vi "fgt set sensor Custom Scale Ex.vi"(8 "error in (no error)":errorcluster, 9 "SMax":sgl, 10 "Custom scale":T1, 11 "sensorIndex":u32) -> (0 "error out":errorcluster)   [LabVIEW 2020, in "fgt_SDK.lvlib"]
doc: "Apply a custom scale factor on sensor read value. This function is useful in order to adapt read sensor value to physical measurement.\nFor example if a flow-unit is used with a special oil and it's calibration table is set to H2O, read flowrate is not correct.\nScale factor is applied using following formula: scaled_value = a*sensor_value + b*sensor_value^2 + c*sensor_value^3.\nWhen applying a custom scale factor, sensor range may increase very rapidly, SMax parameter is ment to limit this maximal value.\nThis function purpose is to be used with the regulation in order to avoid too high maximum range on the sensor. Not supported by IPS."
uses:
  fgt_SDK.lvlib
  TypeDefs/fgt_SCALE.ctl
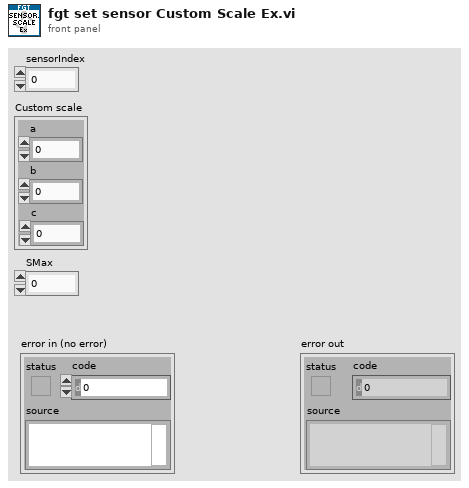
[diagram p1: front panel]
types:
  T1 = typedef "fgt_SDK.lvlib/fgt_SCALE.ctl" = cluster{"a":sgl, "b":sgl, "c":sgl}
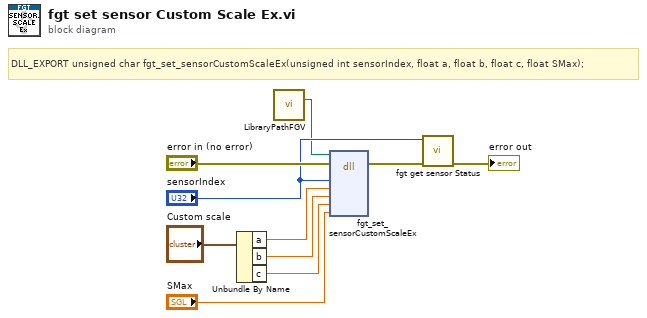
[diagram p0: block diagram]
diagram:
  # "DLL_EXPORT unsigned char fgt_set_sensorCustomScaleEx(unsigned int sensorIndex, float a, float b, float c, float SMax);"
  n1 = Unbundle By Name("Custom scale") -> ("a"=w4:sgl, "b"=w3:sgl, "c"=w2:sgl)
  n2 = call "LibraryPathFGV.vi"() -> ("Path Out"=w1:path)  [unwired: 14 in, 1 out]
  n3 = dll-call lib="C:/Workspace/fgt-SDK/LabVIEW/dlls/fgt_SDK_*.*" fn="fgt_set_sensorCustomScaleEx"(path in=w1, error in="error in (no error)", "sensorIndex"="sensorIndex", "a"=w4, "b"=w3, "c"=w2, "SMax"="SMax") -> (error out=w8:errorcluster)  [unwired: 7 in, 1 out]
  n4 = call "fgt get sensor Status.vi"("error in (no error)"=w8, "pressureIndex"="sensorIndex") -> ("error out"=→"error out":errorcluster)  [unwired: 9 in]
